vi "RunPCDispatch.vi"() -> ()   [LabVIEW 2012]
panel:
  out "code":i32
  out "source":string
  out "status":bool
  out "error out":errorcluster
  out "appended path":path
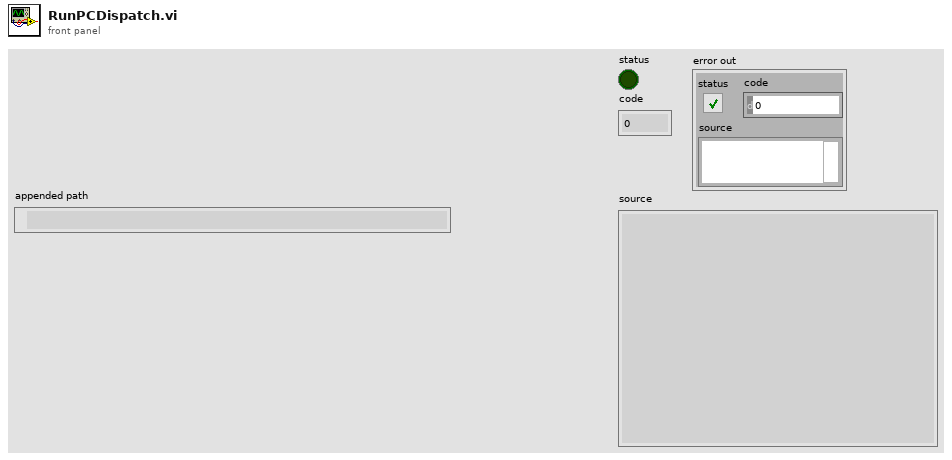
[diagram p1: front panel]
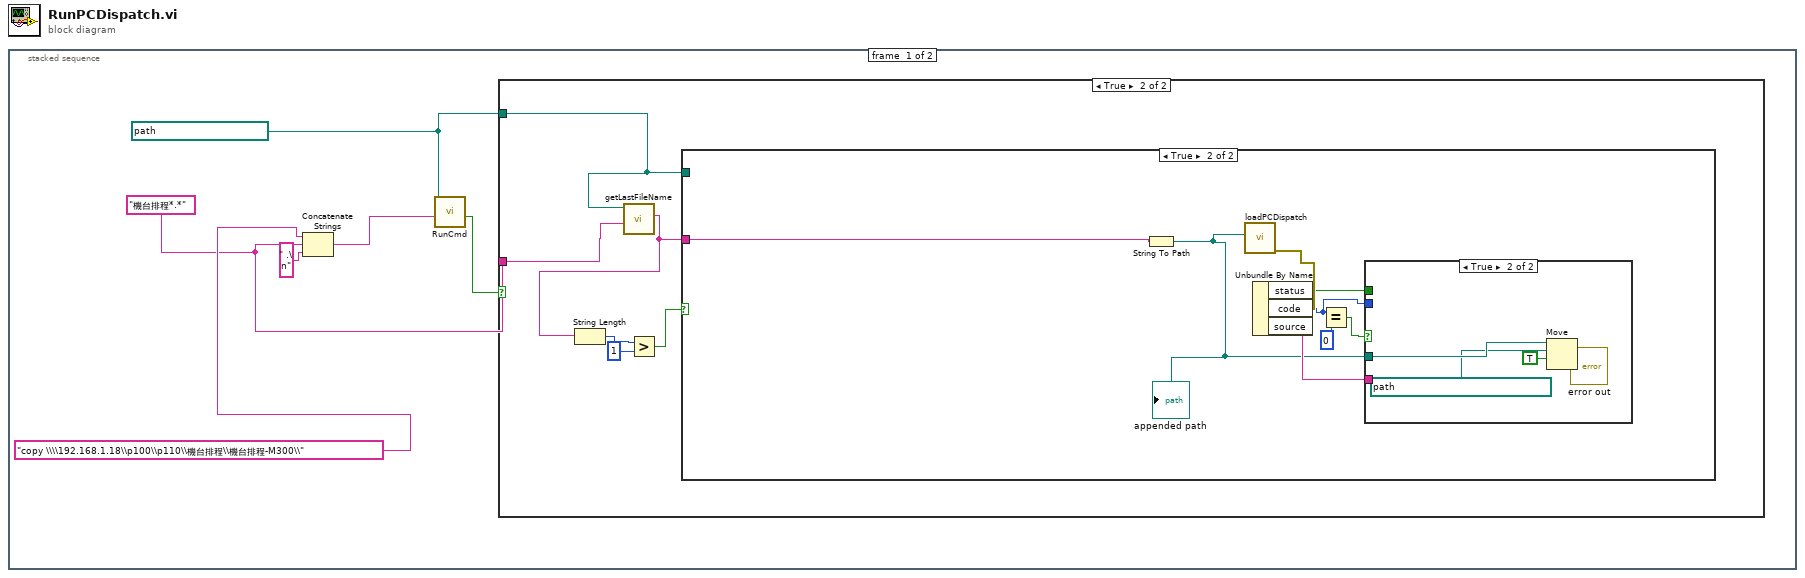
[diagram p0: block diagram]
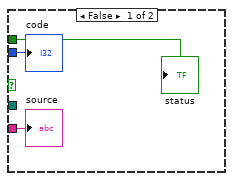
[diagram p4: hidden frame]
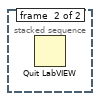
[diagram p5: hidden frame]
diagram:
  n1 = stacked-sequence {
    frame #0 {
      w2 = path "o:/monitor/M300排程" ("path")
      w5 = "機台排程*.*" ("pattern")
      n2 = Concatenate Strings("copy \\\\192.168.1.18\\p100\\p110\\機台排程\\機台排程-M300\\" ("string"), w5, " .\n" ("string")) -> (w3:string)
      n3 = call "RunCmd.vi"("Cmd String"=w3, "working directory"=w2) -> ("OK"=w1:bool)  [unwired: 8 in, 1 out]
      n4 = case shown="True" w1 {
        tunnel: w5 -> [_ w8]
        tunnel: w2 -> [_ w7]
        frame False {
        }
        frame True {
          n5 = call "getLastFileName.vi"("pattern"=w8, "path"=w7) -> ("FileName"=w12:string)  [unwired: 9 in]
          n6 = String Length(string=w12) -> (length=w11:i32)
          n7 = Greater?(x=w11, y=1) -> (0:w9:bool)
          n8 = case shown="True" w9 {
            tunnel: w12 -> [_ w13]
            tunnel: w7 -> [_ _]
            frame False {
            }
            frame True {
              n9 = String To Path(string=w13) -> (path=w14:path)
              "appended path" <- w14
              n10 = call "loadPCDispatch.vi"("template (empty)"=w14) -> ("error out 2"=w20:errorcluster)  [unwired: 10 in]
              n11 = Unbundle By Name(w20) -> ("status"=w17:bool, "code"=w15:i32, "source"=w16:string)
              n12 = Equal?(x=w15, y=0) -> (x = y?=w18:bool)
              n13 = case shown="True" w18 {
                tunnel: w14 -> [_ w27]
                tunnel: w17 -> [w23 _]
                tunnel: w16 -> [w22 _]
                tunnel: w15 -> [w21 _]
                frame False {
                  "status" <- w23
                  "source" <- w22
                  "code" <- w21
                }
                frame True {
                  n14 = Move(source path=w27, 9:TRUE ("overwrite (F)"), 10:path "o:/monitor/M300排程/History" ("path")) -> (error out=→"error out":errorcluster)  [unwired: 2 in, 2 out]
                }
              }
            }
          }
        }
      }
    }
    frame #1 {
      n15 = Quit LabVIEW() -> ()  [unwired: 1 in]
    }
  }
